vi "DBL info.vi"(8 "error in (no error)":errorcluster, 11 "Variant":variant) -> (0 "error out":errorcluster, 3 "child strings":string[](array[string]))   [LabVIEW 2017, in "DSF Mini Explorer.lvlib"]
uses:
  DSF Configuration.llb/DSF Mini Explorer.lvlib
  DSF Configuration.llb/Get Numeric Information.vi
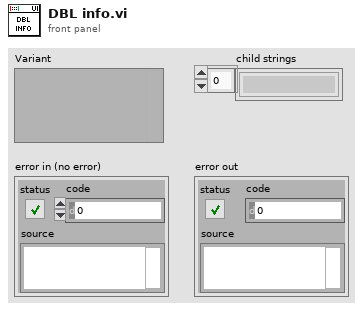
[diagram p1: front panel]
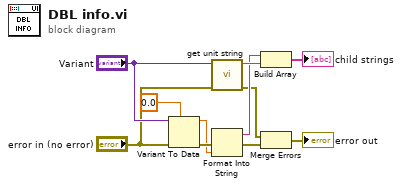
[diagram p0: block diagram]
diagram:
  n1 = Variant To Data(error in="error in (no error)", type=0.0, Variant="Variant") -> (data=w6:dbl, error out=w9:errorcluster)
  n2 = call "get unit string.vi"("error in (no error)"="error in (no error)", "Variant"="Variant") -> ("error out"=w3:errorcluster, "String"=w10:string)  [unwired: 8 in]
  n3 = Format Into String(error in=w9, w6) -> (resulting string=w7:string, error out=w2:errorcluster)  [unwired: 2 in]
  n4 = Build Array(w7, w10) -> (→"child strings":string[])
  n5 = Merge Errors(w3, w2) -> (→"error out":errorcluster)
